vi "in_bounds.vi"(10 "size":dbl=800.0 format="%#_13g", 11 "bbox":T1) -> (3 "bbox_out":cluster{"y":dbl, "y":dbl, "y":dbl, "y":dbl})   [LabVIEW 2024]
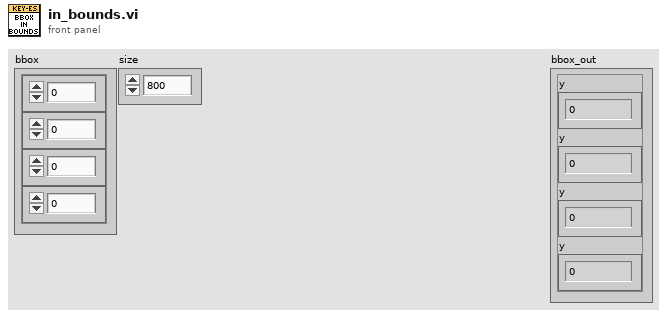
[diagram p1: front panel]
types:
  T1 = cluster{"Numeric Control":dbl, "Numeric Control":dbl, "Numeric Control":dbl, "Numeric Control":dbl}
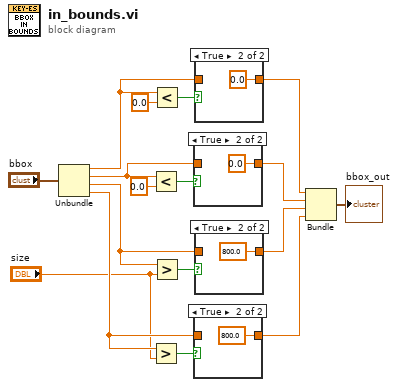
[diagram p0: block diagram]
diagram:
  n1 = Unbundle("bbox") -> ("Numeric Control"=w14:dbl, "Numeric Control"=w11:dbl, "Numeric Control"=w8:dbl, "Numeric Control"=w7:dbl)
  n2 = Less?(x=w11, y=0.0) -> (x < y?=w13:bool)
  n3 = Greater?(x=w7, y="size") -> (0:w10:bool)
  n4 = Less?(x=w14, y=0.0) -> (x < y?=w15:bool)
  n5 = Greater?(x=w8, y="size") -> (0:w9:bool)
  n6 = case shown="True" w13 {
    tunnel: w11 -> [w18 _]
    tunnel: [w18 0.0 ("y")] -> w5
    frame False {
    }
    frame True {
    }
  }
  n7 = case shown="True" w10 {
    tunnel: w7 -> [w20 _]
    tunnel: [w20 800.0 ("y")] -> w2
    frame False {
    }
    frame True {
    }
  }
  n8 = case shown="True" w15 {
    tunnel: w14 -> [w22 _]
    tunnel: [w22 0.0 ("y")] -> w3
    frame False {
    }
    frame True {
    }
  }
  n9 = case shown="True" w9 {
    tunnel: w8 -> [w24 _]
    tunnel: [w24 800.0 ("y")] -> w4
    frame False {
    }
    frame True {
    }
  }
  n10 = Bundle("y"=w3, "y"=w5, "y"=w4, "y"=w2) -> (→"bbox_out":cluster{"y":dbl, "y":dbl, "y":dbl, "y":dbl})  [unwired: 1 in]
